vi "PrintAllTransactions.vi"(7 "Path":path=path "C:/LabViewTesty", 9 "Colors 3":u32[](array[colorbox])=[11796480, 37103, 40712, 16770816, 11796658, 4210752, 15517151], 10 "Transactions:":string[](array[string]), 11 "Pie Chart All Transactions":picture) -> ()   [LabVIEW 2014]
panel:
  out "All transactions":T1={"Pie Chart All Transactions"=bytes[270], "Transactions:"=[], "Colors 3"=[11796480, 37103, 40712, 16770816, 11796658, 4210752, 15517151], "Data"="", "Time"=""}
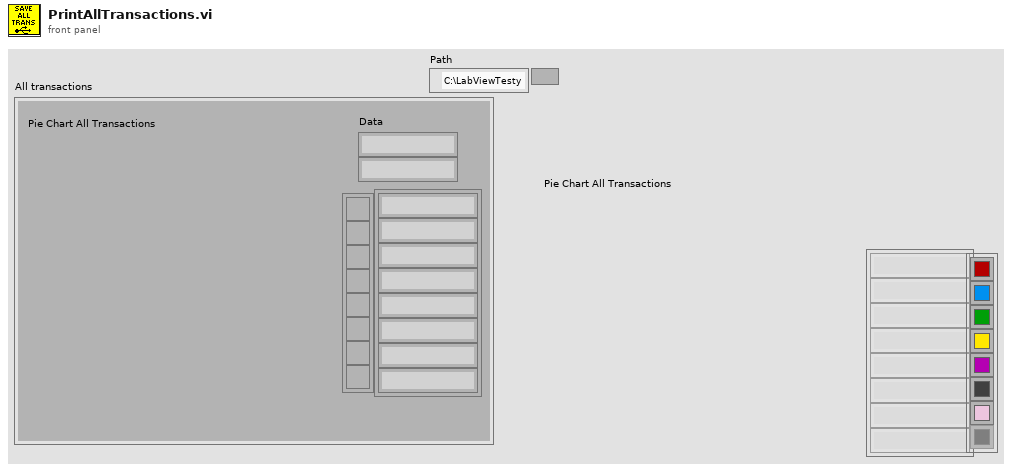
[diagram p1: front panel]
types:
  T1 = cluster{"Pie Chart All Transactions":picture, "Transactions:":string[], "Colors 3":u32[], "Data":string, "Time":string}
  T2 = typedef "imagedata.ctl" = cluster{"image type":i32, "image depth":i32, "image":u8[], "mask":u8[], "colors":u32[], "Rectangle":cluster{"left":i16, "top":i16, "right":i16, "bottom":i16}}
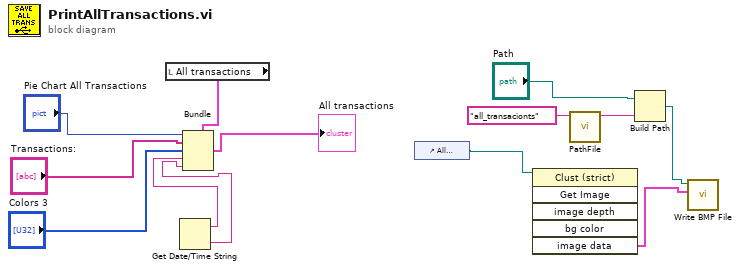
[diagram p0: block diagram]
diagram:
  n1 = local read "All transactions"() -> (w12:T1)
  n2 = Get Date/Time String() -> (date string=w8:string, time string=w7:string)  [unwired: 3 in]
  n3 = Bundle(cluster=w12, "Pie Chart All Transactions"="Pie Chart All Transactions", "Transactions:"="Transactions:", "Colors 3"="Colors 3", "Data"=w8, "Time"=w7) -> (→"All transactions":T1)
  n4 = control-ref of="All transactions"() -> (w1:refnum<vi>)
  n5 = invoke class="Clust (strict)" method="Get Image"(reference=w1) -> ("image data"=w6:T2)  [unwired: 5 in, 5 out]
  n6 = call "PathFile.vi"("NameFile"="all_transacionts") -> ("stringNameFile"=w2:string)  [unwired: 10 in]
  n7 = Build Path(base path="Path", name or relative path=w2) -> (appended path=w5:path)
  n8 = call <vilib>:"Write BMP File.vi"("image data"=w6, "path to BMP file"=w5) -> ()  [unwired: 8 in, 2 out]
